vi "level 1.1.vi"() -> ()   [LabVIEW 2015]
panel:
  out "answer":dbl
  in  "Enum":T1(ring)
  in  "num2 2":dbl
  in  "num1":dbl
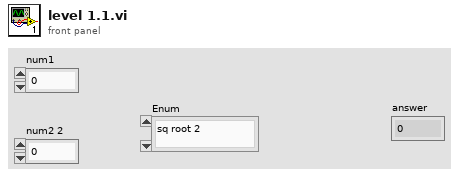
[diagram p1: front panel]
types:
  T1 = enum16{"sq root 2", "sq root 1", "square 2", "square 1", "division", "product", "difference", "sum"}
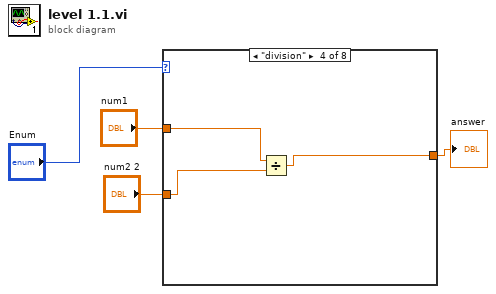
[diagram p0: block diagram]
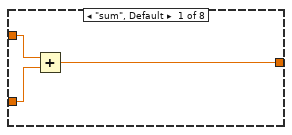
[diagram p2: hidden frame]
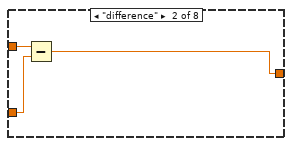
[diagram p3: hidden frame]
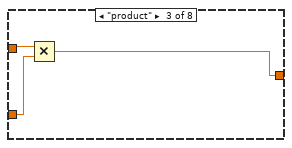
[diagram p4: hidden frame]
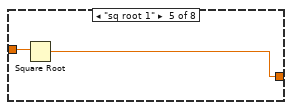
[diagram p5: hidden frame]
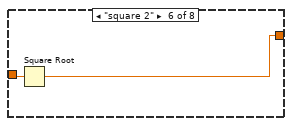
[diagram p6: hidden frame]
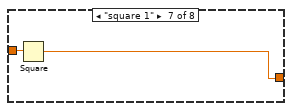
[diagram p7: hidden frame]
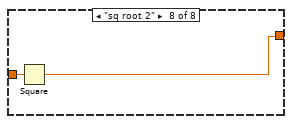
[diagram p8: hidden frame]
diagram:
  n1 = case shown="\"division\"" "Enum" {
    tunnel: "num1" -> [w7 w10 w12 w16 w18 _ w22 _]
    tunnel: "num2 2" -> [w6 w9 w13 w15 _ w19 _ w24]
    tunnel: [w5 w8 w11 w14 w17 w20 w21 w23] -> w1
    frame "sum", Default {
      n2 = Add(x=w7, y=w6) -> (x+y=w5:dbl)
    }
    frame "difference" {
      n3 = Subtract(x=w10, y=w9) -> (x-y=w8:dbl)
    }
    frame "product" {
      n4 = Multiply(x=w12, y=w13) -> (x*y=w11:dbl)
    }
    frame "division" {
      n5 = Divide(x=w16, y=w15) -> (x/y=w14:dbl)
    }
    frame "sq root 1" {
      n6 = Square Root(x=w18) -> (sqrt(x)=w17:dbl)
    }
    frame "square 2" {
      n7 = Square Root(x=w19) -> (sqrt(x)=w20:dbl)
    }
    frame "square 1" {
      n8 = Square(x=w22) -> (x^2=w21:dbl)
    }
    frame "sq root 2" {
      n9 = Square(x=w24) -> (x^2=w23:dbl)
    }
  }
  "answer" <- w1
